vi "VI_ProcessUSerCommands.vi"(8 "error in (no error)":errorcluster, 10 "send command":string, 11 "Common Refs":T1={"LBox_ChList"=refnum, "STR_LoggingChName1"=refnum, "Listbox_ChValue"=refnum, "STR_LoggingChName2"=refnum, "STR_LoggingChName3"=refnum, "STR_LoggingChName4"=refnum, "STR_LoggingChName5"=refnum, "STR_LoggingChName6"=refnum, "OXY_SCPI Ref"="TCPIP0::192.168.1.75::10001::SOCKET", "STR_ChName1"=refnum, "STR_ChName2"=refnum, "STR_ChName3"=refnum, "STR_ChName4"=refnum, "STR_ChName5"=refnum, "STR_ChName6"=refnum, "Enum_SelectTimestampFormat"=refnum, "GRAPH-XY_ELOG"=refnum, "GRAPH-XY_Measurement"=refnum, "Button_StartBuffer"=refnum, "Button_StopBuffer"=refnum, "Button_FetchData"=refnum, "STR_LoggingChName1"=refnum, "STR_LoggingChName2"=refnum, "STR_LoggingChName3"=refnum, "STR_LoggingChName4"=refnum, "STR_LoggingChName5"=refnum, "STR_LoggingChName6"=refnum, "Enum_SelectCalc"=refnum, "Num_SetDurationTime"=refnum, "Button_StopTransfer"=refnum, "Button_StartTransfer"=refnum, "STR_IN_AggregationRate"=refnum, "Button_Disconnect"=refnum, "Button_Connect"=refnum, "Button_StartRec"=refnum, "Button_PauseRec"=refnum, "Button_StopRec"=refnum, "Bool_StatusLED"=refnum, "Indicator_RecordingStatus"=refnum}) -> (0 "error out":errorcluster)   [LabVIEW 2018]
uses:
  TypeDefs/Refs_Common.ctl
  TypeDefs/TD_Case_RecControll_DisableControlls.ctl
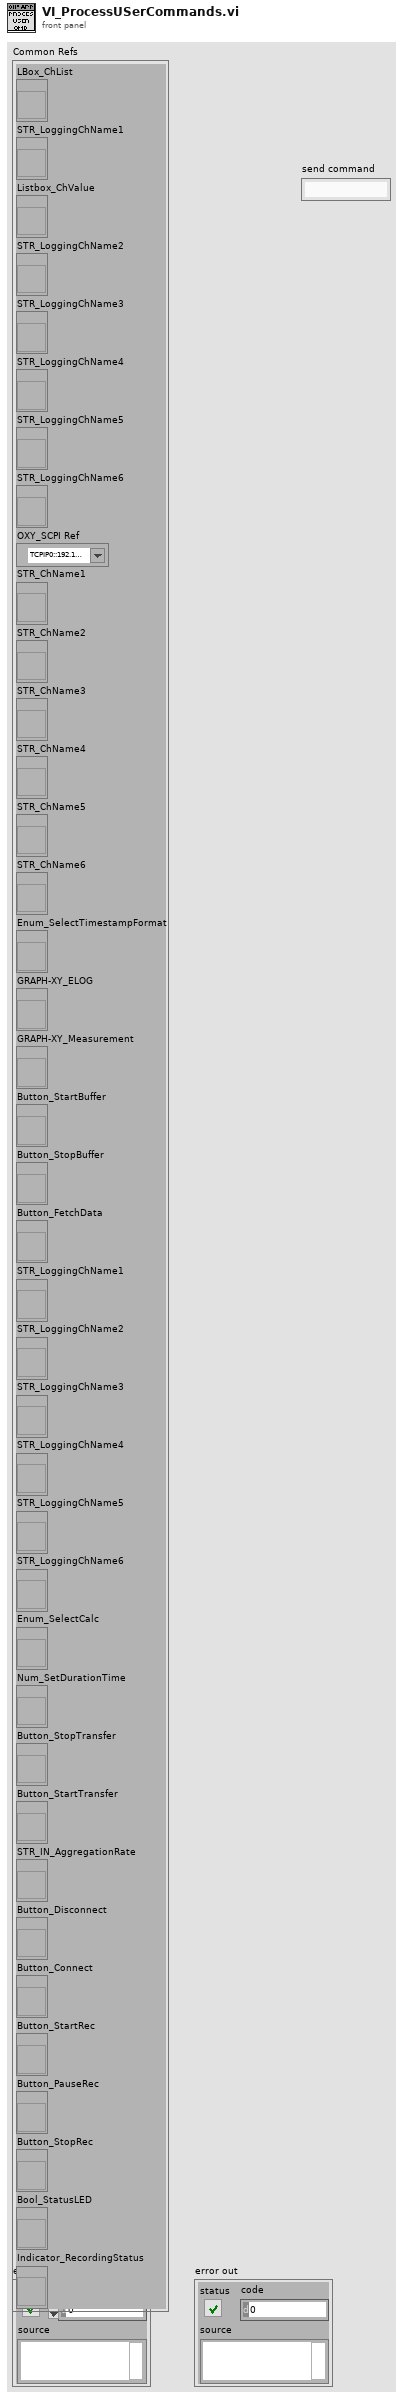
[diagram p1: front panel]
types:
  T1 = typedef "Refs_Common.ctl" = cluster{"LBox_ChList":refnum<vi>, "STR_LoggingChName1":refnum<vi>, "Listbox_ChValue":refnum<vi>, "STR_LoggingChName2":refnum<vi>, "STR_LoggingChName3":refnum<vi>, "STR_LoggingChName4":refnum<vi>, "STR_LoggingChName5":refnum<vi>, "STR_LoggingChName6":refnum<vi>, "OXY_SCPI Ref":refnum<visa-resource-name>, "STR_ChName1":refnum<vi>, "STR_ChName2":refnum<vi>, "STR_ChName3":refnum<vi>, "STR_ChName4":refnum<vi>, "STR_ChName5":refnum<vi>, "STR_ChName6":refnum<vi>, "Enum_SelectTimestampFormat":refnum<vi>, "GRAPH-XY_ELOG":refnum<vi>, "GRAPH-XY_Measurement":refnum<vi>, "Button_StartBuffer":refnum<vi>, "Button_StopBuffer":refnum<vi>, "Button_FetchData":refnum<vi>, "STR_LoggingChName1":refnum<vi>, "STR_LoggingChName2":refnum<vi>, "STR_LoggingChName3":refnum<vi>, "STR_LoggingChName4":refnum<vi>, "STR_LoggingChName5":refnum<vi>, "STR_LoggingChName6":refnum<vi>, "Enum_SelectCalc":refnum<vi>, "Num_SetDurationTime":refnum<vi>, "Button_StopTransfer":refnum<vi>, "Button_StartTransfer":refnum<vi>, "STR_IN_AggregationRate":refnum<vi>, "Button_Disconnect":refnum<vi>, "Button_Connect":refnum<vi>, "Button_StartRec":refnum<vi>, "Button_PauseRec":refnum<vi>, "Button_StopRec":refnum<vi>, "Bool_StatusLED":refnum<vi>, "Indicator_RecordingStatus":refnum<vi>}
  T2 = typedef "TD_Case_RecControll_DisableControlls.ctl" = enum16{"Start", "Pause", "Stop"}
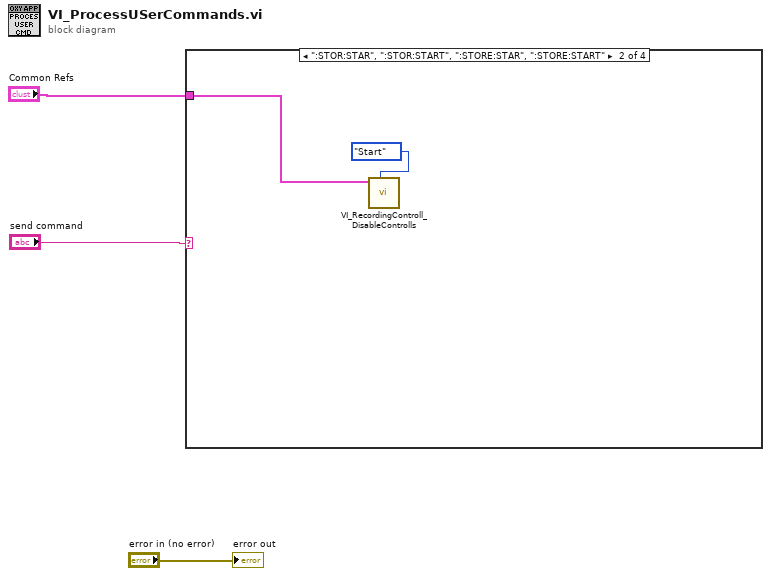
[diagram p0: block diagram]
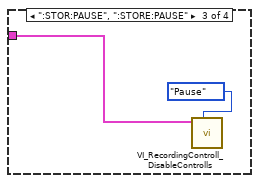
[diagram p3: hidden frame]
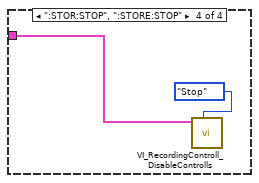
[diagram p4: hidden frame]
diagram:
  n1 = case shown="\":STOR:STAR\", \":STOR:START\", \":STORE:STAR\", \":STORE:START\"" "send command" {
    tunnel: "Common Refs" -> [_ w4 w6 w8]
    frame Default {
    }
    frame ":STOR:STAR", ":STOR:START", ":STORE:STAR", ":STORE:START" {
      n2 = call "VI_RecordingControll_DisableControlls.vi"("Mode"=TD_Case_RecControll_DisableControlls."Start", "Common Refs"=w4) -> ()  [unwired: 9 in, 1 out]
    }
    frame ":STOR:PAUSE", ":STORE:PAUSE" {
      n3 = call "VI_RecordingControll_DisableControlls.vi"("Mode"=TD_Case_RecControll_DisableControlls."Pause", "Common Refs"=w6) -> ()  [unwired: 9 in, 1 out]
    }
    frame ":STOR:STOP", ":STORE:STOP" {
      n4 = call "VI_RecordingControll_DisableControlls.vi"("Mode"=TD_Case_RecControll_DisableControlls."Stop", "Common Refs"=w8) -> ()  [unwired: 9 in, 1 out]
    }
  }
  "error out" <- "error in (no error)"
